vi "Arm and Fire Transient.vi"(8 "error in":errorcluster) -> (0 "error out":errorcluster)   [LabVIEW 2017, in "DTACQ - Network Enabled Device Driver.lvlib"]
doc: "Arms and fires a transient shot. Waits until data is ready for downoad, before exiting the VI."
uses:
  DTACQ - Network Enabled Device Driver.lvlib
  Communications/Typedefs/DTACQ Status--Enum.ctl
  Communications/Typedefs/Functional Global Variable Action--Enum.ctl
  Communications/Communications Library.lvlib
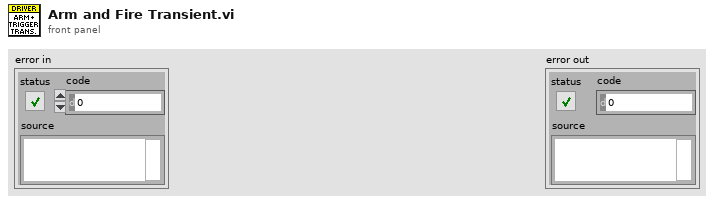
[diagram p1: front panel]
types:
  T1 = typedef "Communications Library.lvlib/Functional Global Variable Action--Enum.ctl" = enum16{"Initialise", "Write Module Config", "Write Carrier Config", "Read"}
  T2 = typedef "Communications Library.lvlib/DTACQ Module Carrier Configuration--Cluster.ctl" = cluster{"Name":string, "IP":string, "Control Port":i32, "Timeout (ms)":i32, "Continuous Capture Port (Multiplexed)":i32, "Start HIL Shot Port":i32, "AWG Upload Port (Multiplexed)":i32, "Download Captured Data Port (Multiplexed)":i32, "Module Slots":i32, "Module Configurations":T3[]}
  T3 = typedef "Communications Library.lvlib/DTACQ Module Configuration--Cluster.ctl" = cluster{"Name":string, "Position":string, "Module Type":T4, "Control Port":i32, "Timeout (ms)":i32, "Channels":i32}
  T4 = typedef "Communications Library.lvlib/DTACQ Device Type--Enum.ctl" = enum16{"Carrier", "Analog In Module", "Analog Out Module", "Generic Module"}
  T5 = typedef "Communications Library.lvlib/DTACQ Connection Data--Cluster.ctl" = cluster{"Description":string, "Address":string, "Port":u16, "timeout (ms)":i32, "Termination Character":string, "TCP Connection Reference":refnum<k5>, "Open Connection":bool}
  T6 = typedef "Communications Library.lvlib/DTACQ Status--Enum.ctl" = enum16{"IDLE", "ARM", "RUN_PRE-TRIGGER", "RUN_POST-TRIGGER", "POST_PROCESS", "CLEANUP"}
  T7 = typedef "Communications Library.lvlib/DTACQ Module Carrier Status.ctl" = cluster{"DTACQ State":T6, "Pre-Trigger Samples":i32, "Post-Trigger Samples":i32, "Total Samples":i32, "Post Processing":bool}
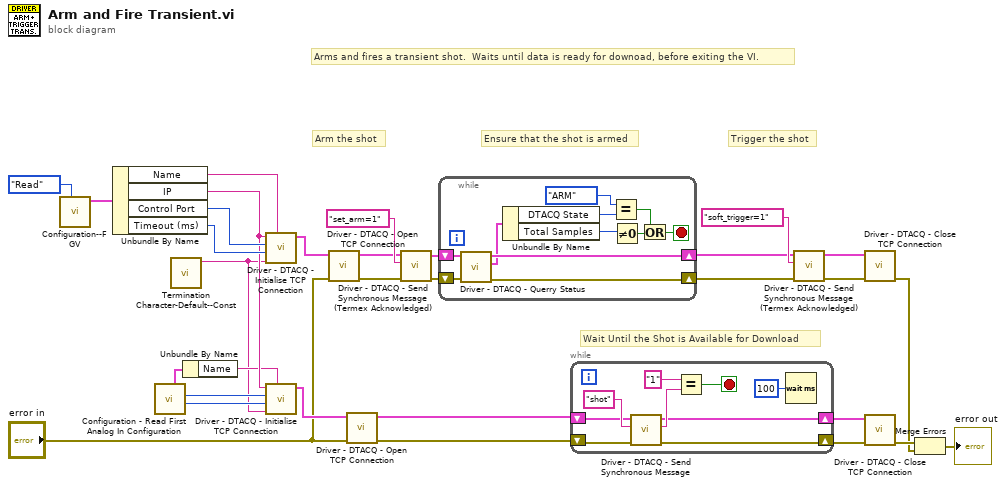
[diagram p0: block diagram]
diagram:
  # "Arms and fires a transient shot.  Waits until data is ready for downoad, before exiting the VI."
  # "Ensure that the shot is armed"
  # "Trigger the shot"
  # "Arm the shot"
  # "Wait Until the Shot is Available for Download"
  n1 = call "Configuration--FGV.vi"("Functional Global Action"=Functional_Global_Variable_Action--Enum."Read") -> ("Carrier Configuration Out"=w24:T2)  [unwired: 9 in, 1 out]
  n2 = Unbundle By Name(w24) -> ("Name"=w23:string, "IP"=w18:string, "Control Port"=w22:i32, "Timeout (ms)"=w21:i32)
  n3 = call "Configuration - Read First Analog In Configuration.vi"() -> ("Timeout (ms)"=w20:i32, "Analog In Control Port"=w19:i32, "AI - Module Configuration"=w17:T3)  [unwired: 7 in, 2 out]
  n4 = call "Termination Character-Default--Const.vi"() -> ("Termination Character"=w14:string)  [unwired: 11 in]
  n5 = Unbundle By Name(w17) -> ("Name"=w16:string)
  n6 = call "Driver - DTACQ - Initialise TCP Connection.vi"("Description"=w23, "Termination Character"=w14, "timeout (ms)"=w21, "Port"=w22, "Address"=w18) -> ("DTACQ Connection Data Out"=w26:T5)  [unwired: 6 in]
  n7 = call "Driver - DTACQ - Initialise TCP Connection.vi"("Description"=w16, "Termination Character"=w14, "timeout (ms)"=w20, "Port"=w19, "Address"=w18) -> ("DTACQ Connection Data Out"=w15:T5)  [unwired: 6 in]
  n8 = call "Driver - DTACQ - Open TCP Connection.vi"("error in"="error in", "DTACQ Connection Data In"=w26) -> ("error out"=w27:errorcluster, "DTACQ Connection Data Out"=w28:T5)  [unwired: 8 in]
  n9 = call "Driver - DTACQ - Open TCP Connection.vi"("error in"="error in", "DTACQ Connection Data In"=w15) -> ("error out"=w12:errorcluster, "DTACQ Connection Data Out"=w13:T5)  [unwired: 8 in]
  n10 = call "Driver - DTACQ - Send Synchronous Message (Termex Acknowledged).vi"("error in"=w27, "Message to Send"="set_arm=1", "DTACQ Connection Data In"=w28) -> ("error out"=w31:errorcluster, "DTACQ Connection Data Out"=w30:T5)  [unwired: 5 in, 2 out]
  n11 = while {
    shift-right: [w39] -> w9
    shift-left: w30 -> [w41]
    shift-right: [w40] -> w10
    shift-left: w31 -> [w42]
    stop <- w32 stop-if-true
    n12 = call "Driver - DTACQ - Querry Status.vi"("error in"=w42, "DTACQ Connection Data In"=w41) -> ("error out"=w40:errorcluster, "Module Carrier Status"=w38:T7, "DTACQ Connection Data Out"=w39:T5)  [unwired: 6 in, 1 out]
    n13 = Unbundle By Name(w38) -> ("DTACQ State"=w37:T6, "Total Samples"=w35:i32)
    n14 = Equal?(x=DTACQ_Status--Enum."ARM", y=w37) -> (x = y?=w33:bool)
    n15 = Not Equal To 0?(x=w35) -> (x != 0?=w34:bool)
    n16 = Or(x=w33, y=w34) -> (x .or. y?=w32:bool)
  }
  n17 = while {
    shift-right: [w46] -> w5
    shift-left: w12 -> [w48]
    shift-right: [w45] -> w6
    shift-left: w13 -> [w47]
    stop <- w44 stop-if-true
    n18 = call "Driver - DTACQ - Send Synchronous Message.vi"("error in"=w48, "Message to Send"="shot", "DTACQ Connection Data In"=w47) -> ("error out"=w46:errorcluster, "Read String"=w49:string, "DTACQ Connection Data Out"=w45:T5)  [unwired: 5 in, 1 out]
    n19 = Equal?(x="1" ("y"), y=w49) -> (x = y?=w44:bool)
    n20 = Wait (ms)(milliseconds to wait=u32 100) -> ()  [unwired: 1 out]
  }
  n21 = call "Driver - DTACQ - Send Synchronous Message (Termex Acknowledged).vi"("error in"=w10, "Message to Send"="soft_trigger=1", "DTACQ Connection Data In"=w9) -> ("error out"=w7:errorcluster, "DTACQ Connection Data Out"=w8:T5)  [unwired: 5 in, 2 out]
  n22 = call "Driver - DTACQ - Close TCP Connection.vi"("error in"=w7, "DTACQ Connection Data In"=w8) -> ("error out"=w2:errorcluster)  [unwired: 8 in, 1 out]
  n23 = call "Driver - DTACQ - Close TCP Connection.vi"("error in"=w5, "DTACQ Connection Data In"=w6) -> ("error out"=w3:errorcluster)  [unwired: 8 in, 1 out]
  n24 = Merge Errors(w3, w2) -> (→"error out":errorcluster)
